vi "GetFrontPanel.vi"(8 "ErrorIn":errorcluster, 11 "ReferenceIn":refnum<class "JSONTextViewer.lvclass">) -> (0 "ErrorOut":errorcluster, 2 "FrontPanel":refnum<class "FrontPanelControl.lvclass">, 3 "ReferenceOut":refnum<class "JSONTextViewer.lvclass">)   [LabVIEW 2021, in "JSONTextViewer.lvlib" / "JSONTextViewer.lvclass"]
uses:
  JSONTextViewer.lvclass
  .Externals/Library_UserInterface_FrontPanelControl/FrontPanelControl/FrontPanelControl.lvclass
  JSONTextViewer.lvclass/JSONTextViewer.ctl
  C:/Localdata/Projects/TriekselSoft/TriekselsoftApplicationFramework/Source/.Externals/Library_TAF_ApplicationFramework/TAFBaseGUI/TAFBaseGUI.lvclass
  C:/Localdata/Projects/TriekselSoft/TriekselsoftApplicationFramework/Source/.Externals/Interface_UserInterface_IFrontPanel/IFrontPanel/IFrontPanel.lvclass
  C:/Localdata/Projects/TriekselSoft/TriekselsoftApplicationFramework/Source/IInterface/IInterface.lvclass
  C:/Localdata/Projects/TriekselSoft/TriekselsoftApplicationFramework/Source/.Externals/Interface_TAF_ITAFGUIActions/ITAFGUIActions/ITAFGUIActions.lvclass
  C:/Localdata/Projects/TriekselSoft/TriekselsoftApplicationFramework/Source/.Externals/Interface_TAF_ITextViewer/ITAFTextViewer.lvclass
  C:/Localdata/Projects/TriekselSoft/TriekselsoftApplicationFramework/Source/.Externals/Interface_Object_ICreateDestroy/ICreateDestroy/ICreateDestroy.lvclass
  C:/Localdata/Projects/TriekselSoft/TriekselsoftApplicationFramework/Source/.Externals/Interface_Object_IPersistentData/IPersistentData/IPersistentData.lvclass
  C:/Localdata/Projects/TriekselSoft/TriekselsoftApplicationFramework/Source/.Externals/Interface_TAF_ITAFObject/ITAFObject/ITAFObject.lvclass
  C:/Localdata/Projects/TriekselSoft/TriekselsoftApplicationFramework/Source/ActiveObjects/JSONTextViewer/JSONTextViewer/JSONTextViewer.lvclass
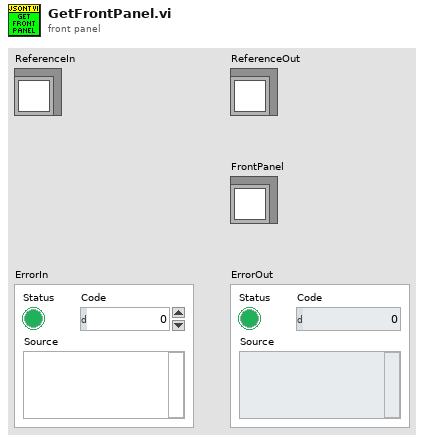
[diagram p1: front panel]
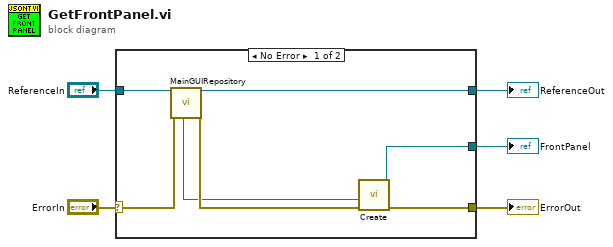
[diagram p0: block diagram]
diagram:
  n1 = case shown="No Error" "ErrorIn" {
    selector: "ErrorIn" -> [w12 w14]
    tunnel: [w10 w14] -> w4
    tunnel: [w8 w13] -> w2
    tunnel: "ReferenceIn" -> [w9 w13]
    tunnel: [w6 _] -> w1
    frame No Error {
      n2 = call "MainGUIRepository.vi"("ReferenceIn"=w9, "ErrorIn"=w12) -> ("ProcessViRef"=w7:refnum<vi>, "ReferenceOut"=w8:refnum<class "JSONTextViewer.lvclass">, "ErrorOut"=w11:errorcluster)  [unwired: 10 in, 5 out]
      n3 = call "Create.vi"("ErrorIn"=w11, "VIRef"=w7) -> ("ErrorOut"=w10:errorcluster, "ObjectOut"=w6:refnum<class "FrontPanelControl.lvclass">)  [unwired: 8 in]
    }
    frame Error {
    }
  }
  "ErrorOut" <- w4
  "ReferenceOut" <- w2
  "FrontPanel" <- w1
